vi "UI-Main.vi"() -> ()   [LabVIEW 2014]
panel:
  out "错误输出":errorcluster
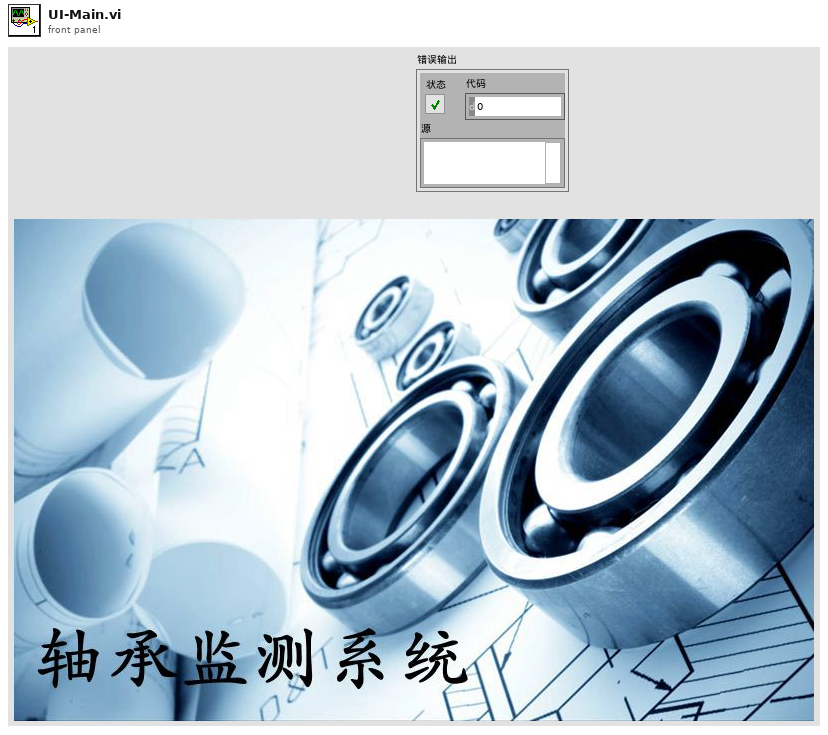
[diagram p1: front panel]
types:
  T1 = enum32{"Invalid", "Standard", "Closed", "Hidden", "Minimized", "Maximized"}
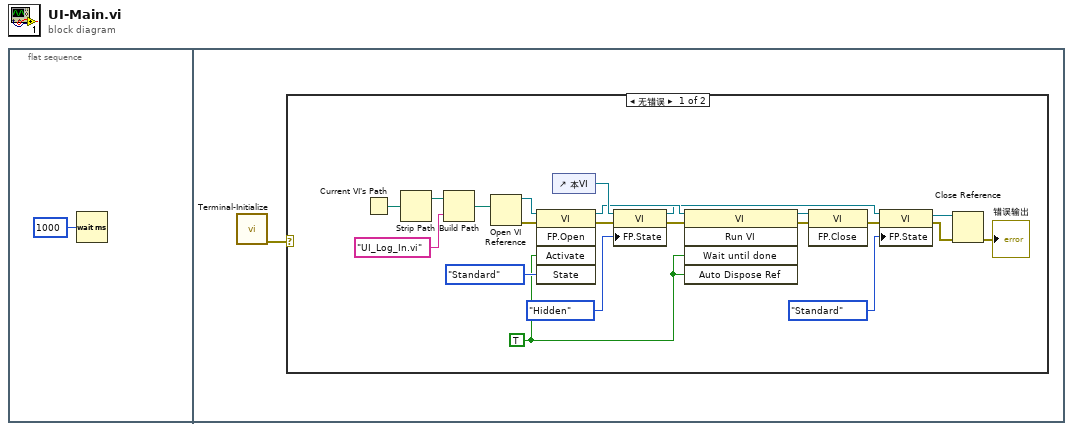
[diagram p0: block diagram]
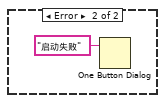
[diagram p2: hidden frame]
diagram:
  n1 = flat-sequence {
    frame #0 {
      n2 = Wait (ms)(milliseconds to wait=u32 1000 ("等待时间（毫秒）")) -> ()  [unwired: 1 out]
    }
    frame #1 {
      n3 = call "Terminal-Initialize.vi"() -> ("error IO"=w2:errorcluster)  [unwired: 11 in]
      n4 = case shown="无错误" w2 {
        frame No Error {
          w6 = TRUE ("激活？")
          n5 = Current VI's Path() -> (path=w22:path)
          n6 = Strip Path(path=w22) -> (stripped path=w21:path)  [unwired: 1 out]
          n7 = Build Path(base path=w21, name or relative path="UI_Log_In.vi" ("名称或相对路径")) -> (appended path=w23:path)
          n8 = Open VI Reference(vi path=w23) -> (vi reference=w19:refnum<vi>, error out=w18:errorcluster)  [unwired: 5 in]
          n9 = invoke class="VI" method="FP.Open"(reference=w19, error in=w18, "Activate"=w6, "State"=T1."Standard" ("状态")) -> (reference out=w10:refnum<vi>, error out=w13:errorcluster)  [unwired: 1 in, 3 out]
          n10 = control-ref of="本VI"() -> (w14:refnum<vi>)
          n11 = property class="VI"(reference=w14, error in=w13, "FP.State"=T1."Hidden" ("前面板窗口:状态")) -> (reference out=w9:refnum<vi>, error out=w11:errorcluster)
          n12 = invoke class="VI" method="Run VI"(reference=w10, error in=w11, "Wait until done"=w6, "Auto Dispose Ref"=w6) -> (reference out=w16:refnum<vi>, error out=w15:errorcluster)  [unwired: 1 in, 3 out]
          n13 = invoke class="VI" method="FP.Close"(reference=w16, error in=w15) -> (error out=w8:errorcluster)  [unwired: 1 in, 2 out]
          n14 = property class="VI"(reference=w9, error in=w8, "FP.State"=T1."Standard" ("前面板窗口:状态")) -> (reference out=w5:refnum<vi>, error out=w4:errorcluster)
          n15 = Close Reference(reference=w5, error in (no error)=w4) -> (error out=→"错误输出":errorcluster)
        }
        frame Error {
          n16 = One Button Dialog(message="启动失败" ("消息")) -> ()  [unwired: 1 in, 1 out]
        }
      }
    }
  }
